vi "Update All Data.vi"(8 "error in (no error)":errorcluster, 10 "Item Names":string[][](array[string]), 11 "MCLB_Lib in":refnum<class "MCLB_Lib.lvclass">) -> (0 "error out":errorcluster, 3 "MCLB_Lib out":refnum<class "MCLB_Lib.lvclass">)   [LabVIEW 2020, in "MCLB_Lib.lvclass"]
uses:
  MCLB_Lib.lvclass
  MCLB_Lib.lvclass/MCLB_Lib.ctl
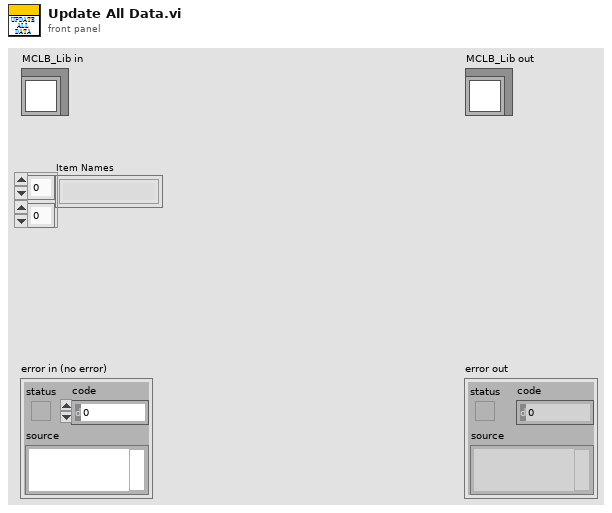
[diagram p1: front panel]
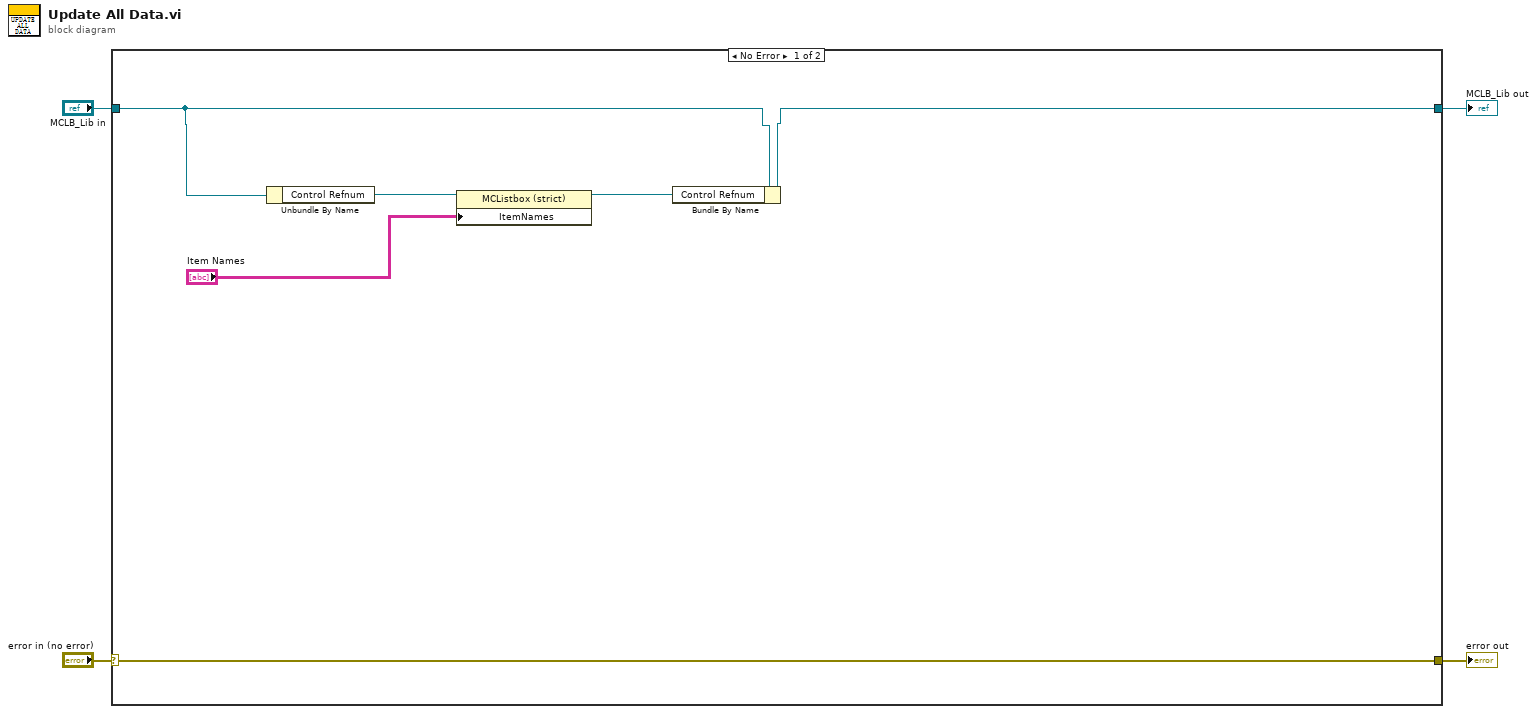
[diagram p0: block diagram]
diagram:
  n1 = case shown="No Error" "error in (no error)" {
    selector: "error in (no error)" -> [w10 w12]
    tunnel: [w10 w12] -> w3
    tunnel: [w7 w11] -> w1
    tunnel: "MCLB_Lib in" -> [w6 w11]
    frame No Error {
      n2 = Unbundle By Name(w6) -> ("Control Refnum"=w8:refnum<vi>)
      n3 = property class="MCListbox (strict)"(reference=w8, "ItemNames"="Item Names") -> (reference out=w9:refnum<vi>)  [unwired: 1 in, 1 out]
      n4 = Bundle By Name(cluster=w6, "Control Refnum"=w9) -> (w7:refnum<class "MCLB_Lib.lvclass">)
    }
    frame Error {
    }
  }
  "error out" <- w3
  "MCLB_Lib out" <- w1
